vi "PDF_Interface_PDF Protokoll HangUp.vi"(8 "error in (no error)":errorcluster caption="Fehler (Eingang, kein Fehler)", 11 "Save PDF File Path":path) -> (0 "error out":errorcluster caption="Fehler (Ausgang)")   [LabVIEW 2020, in "Hangup Check.lvlib"]
uses:
  Hangup Check.lvlib
  Sprachverwaltung/FGV Aktion Tabelle zerlegen.ctl
  AktionFGV Hangup.ctl
  Seiten/System Einstellungen V2/Aktioen FGV System Konstanten.ctl
  PDF_Interface/PDF Protokoll Standard Kopf Optionen.ctl
  <vilib>/Simplicity AI/SAI_PDF_API/Classes/Context/Controls/SAI_PDF_PDF Details.ctl
  PDF_Interface/PDF Interface Helper/PDFContentType.ctl
  PDF_Interface/PDF Interface Helper/PDFTableContentType.ctl
  PDF_Interface/PDF Interface Helper/PDFResults.ctl
  PDF_Interface/PDF Interface Helper/PDFResultPictures.ctl
  PDF_Interface/PDF Interface Helper/PDFCommentPosition.ctl
  PDF_Interface/PDF Interface Helper/PDFPageBreak.ctl
  PDF_Interface/PDF Interface Helper/PDFTablePictures.ctl
  PDF_Interface/PDF Interface Helper/PDFBemerkung.ctl
  <vilib>/Simplicity AI/SAI_PDF_API/Classes/Context/Controls/SAI_PDF_Text Align.ctl
  <vilib>/Simplicity AI/SAI_PDF_API/Classes/Context/Controls/SAI_PDF_Font.ctl
  <vilib>/Simplicity AI/SAI_PDF_API/Classes/Context/Controls/SAI_PDF_Font Encoding.ctl
  Allgemein/allgemeine Sub-VIs.lvlib
  Seiten/System Einstellungen V2/System Einstellungen V2.lvlib
  Sprachverwaltung/Sprachverwaltung.lvlib
  PDF_Interface/PDF Interface.lvlib
  <vilib>/Simplicity AI/SAI_PDF_API/Classes/Context/Context.lvclass
  PDF_Interface/PDF Interface Helper/PDF Interface Helper.lvlib
  Linearisierung V2/Protokoll/Protokoll.lvlib
panel:
  out "Bestanden":bool caption="Boolesch"
  out "Grenzwert:":string
  out "Nullgas Messwert:":string
  out "Datenerfassungszeit:":string
  out "Nullgas Aufschaltzeit:":string
  out "Analysator:":string
  out "Aufschaltpunkt:":string
  out "Messbereich:":string
  out "Endzeit:":string
  out "Startzeit:":string
  out "Ser.Nr.:":string caption="Serien Nummer:"
  out "Messgerät:":string
  # "Hang - up Check"
  # "ppm"
  # "s"
  # "s"
  # "ppmC3"
  # "ppmC3"
  # "IAG-Industrie Automatisierungsgeschellschaft m.b.H.    l  Industriestraße 2    l    2722Weikersdorf     )+43262221734 7+43262221734655"
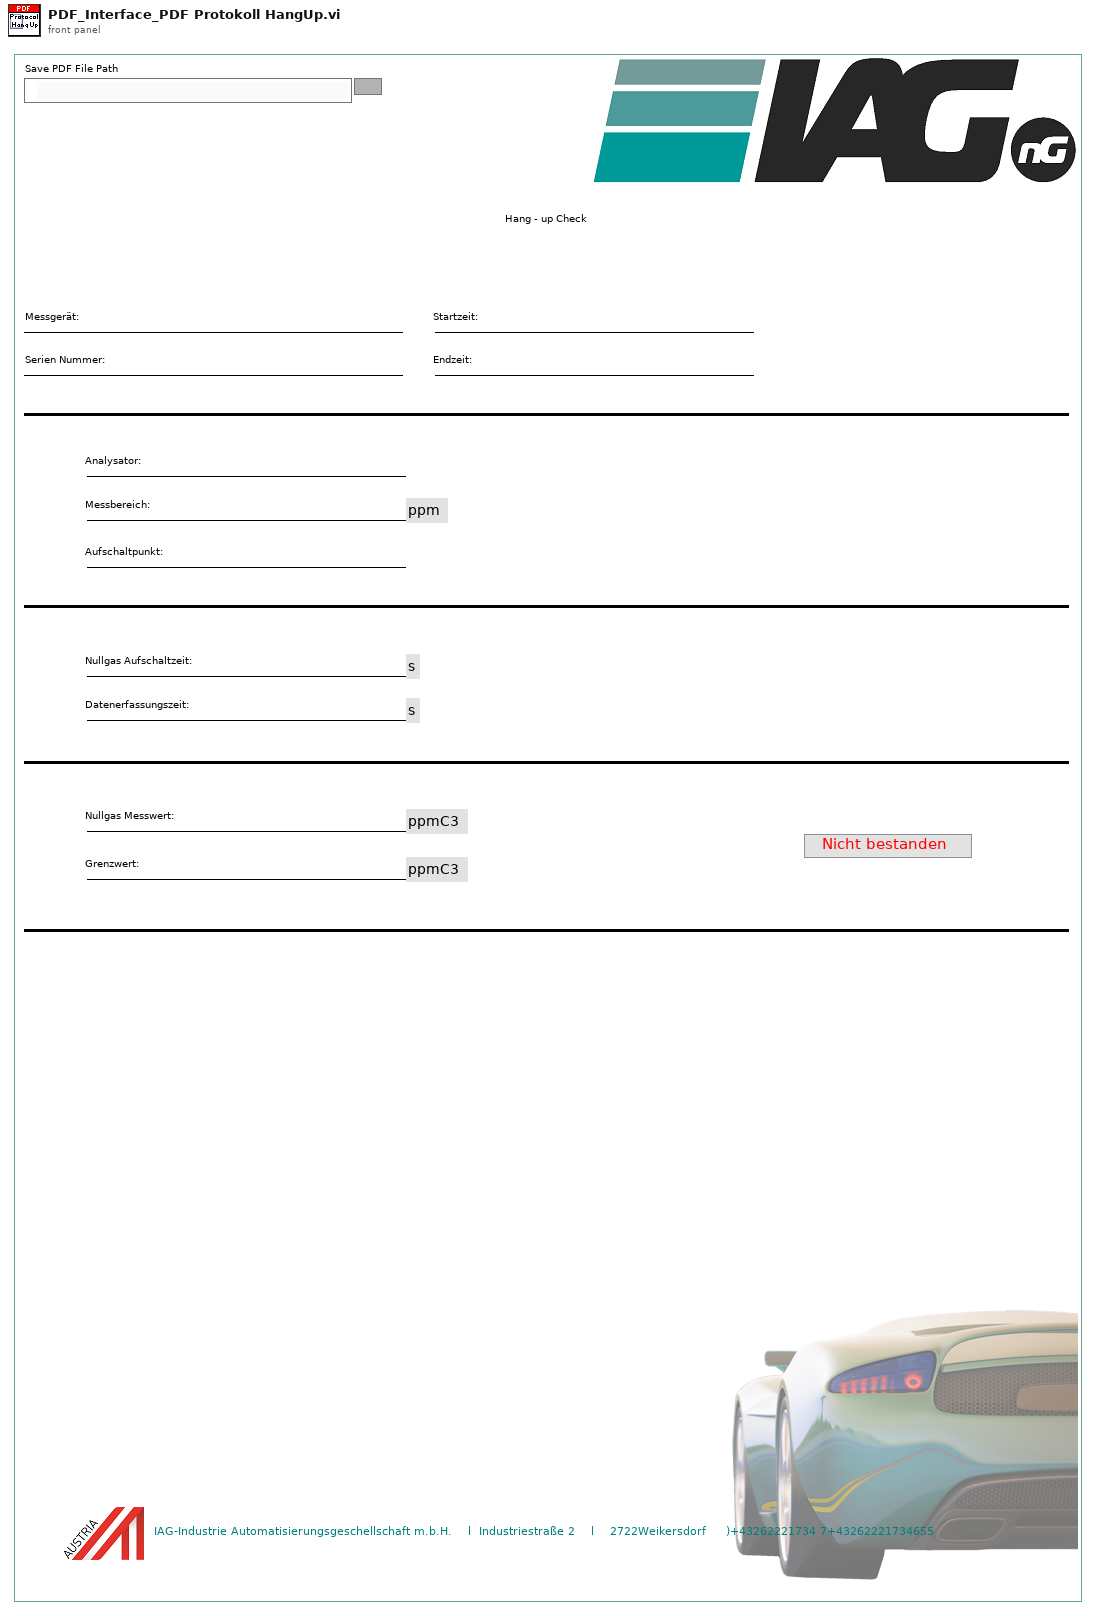
[diagram p1: front panel]
types:
  T1 = typedef "Sprachverwaltung.lvlib/FGV Aktion Tabelle zerlegen.ctl" = enum16{"laden", "vereinzeln", "speichern"}
  T2 = typedef "PDF Interface.lvlib/PDF Protokoll Standard Kopf Optionen.ctl" = cluster{"Analysator":bool, "FT-IR Rezept":bool, "Gasteiler":bool, "Gas Komponente":bool, "Gas Flasche":bool, "LIN Protokoll":bool, "Operator":bool}
  T3 = typedef "System Einstellungen V2.lvlib/Aktioen FGV System Konstanten.ctl" = enum16{"lesen", "laden", "speichern", "Sprache"}
  T4 = typedef "Hangup Check.lvlib/AktionFGV Hangup.ctl" = enum16{"lesen", "Hangup Settings", "Protokoll", "Pfad", "laden", "speichern"}
  T5 = typedef "PDF Interface.lvlib/PDF Interface Helper.lvlib/PDFBemerkung.ctl" = cluster{"Bemerkung Text":string, "Align (Left)":T6, "Add Line Feeds (F:No)":bool, "Font":T7}
  T6 = typedef "SAI_PDF_Toolkit.lvlib/Context.lvclass/SAI_PDF_Text Align.ctl" = i32
  T7 = typedef "SAI_PDF_Toolkit.lvlib/Context.lvclass/SAI_PDF_Font.ctl" = cluster{"Font":string, "Size":i32, "Colour":u32, "Bold":bool, "Italic":bool, "Underline":bool, "Strikethrough":bool, "Font Encoding":T8}
  T8 = typedef "SAI_PDF_Toolkit.lvlib/Context.lvclass/SAI_PDF_Font Encoding.ctl" = enum16{"Cp1252, WinANSI", "IdentityH", "IdentityV", "Cp1250", "Cp1257", "MacRoman"}
  T9 = typedef "PDF Interface.lvlib/PDF Interface Helper.lvlib/PDFResults.ctl" = cluster{"Results":cluster{"Result Text":string, "Result":bool}[], "ResultPictures":T10, "use Pictures":bool, "Image Scale (%)":sgl, "Autoscale? (T)":bool, "Horizontal Align":i32, "Position":i32}
  T10 = typedef "PDF Interface.lvlib/PDF Interface Helper.lvlib/PDFResultPictures.ctl" = cluster{"Yes Ctl Refnum":refnum<vi>, "No Ctl Refnum":refnum<vi>}
  T11 = typedef "PDF Interface.lvlib/PDF Interface Helper.lvlib/PDFTableContentType.ctl" = cluster{"TableHeader":string[], "Table":string[][], "Relative Column Widths (%)":sgl[], "Results":T9, "PositionBemerkung":T12, "PageBreak":T13, "TablePictures":T14, "Horizontal Align":i32}
  T12 = typedef "PDF Interface.lvlib/PDF Interface Helper.lvlib/PDFCommentPosition.ctl" = enum16{"before", "after"}
  T13 = typedef "PDF Interface.lvlib/PDF Interface Helper.lvlib/PDFPageBreak.ctl" = enum16{"none", "before", "after", "after comment"}
  T14 = typedef "PDF Interface.lvlib/PDF Interface Helper.lvlib/PDFTablePictures.ctl" = cluster{"Ctl Refnum In":refnum<vi>[], "RowOrColumn":enum16{"Row", "Column"}, "IndexToInsert":u16, "Image Scale (%)":sgl[], "Autoscale? (T)":bool[], "Horizontal Align":i32}
  T15 = typedef "PDF Interface.lvlib/PDF Interface Helper.lvlib/PDFContentType.ctl" = cluster{"Titel":string, "Header Table":string[][], "Table Array":T11[], "Bemerkungen":T5[]}
  T16 = typedef "SAI_PDF_Toolkit.lvlib/Context.lvclass/SAI_PDF_PDF Details.ctl" = cluster{"Title":string, "Subject":string, "Keywords":string, "Author":string, "Creator":string}
  T17 = cluster{"Header Footer Text Cluster":cluster{"Header Text":string, "Footer Text":string, "Time":string, "Page Number":string}, "PDF Details":T16}
  T18 = typedef "Hangup Check.lvlib/HangupSettings.ctl" = cluster{"Kalibriergas":T19, "Aufschaltpunkt":T19, "Spangas Aufschaltzeit:":sgl, "Nullgas Aufschaltzeit:":sgl, "Datenerfassungszeit:":sgl, "Grenzwert manuell:":sgl, "Grenzwert:":sgl, "Grenze":T19, "Messbereich":T19, "Spankonzentration [ppm]":sgl, "Grenzwert: C1":sgl}
  T19 = typedef "Auswahlfeld.ctl" = u16
  T20 = typedef "Hangup Check.lvlib/Protokoll.ctl" = cluster{"FID Mittelwert 0":sgl, "FID Mittelwert E":sgl, "Messgasdruck Amium":sgl, "Startzeit":timestamp, "Endzeit":timestamp, "Bestanden?":bool}
  T21 = cluster{"Modell":string, "ProjektNummer":string, "Software Version":string, "Seriennummer":string}
  T22 = cluster{"Header Size":i32, "Column Ratio left":sgl[]}
  T23 = typedef "String - Ausgabefeld.ctl" = string
  T24 = cluster{"String - Ausgabefeld":T23, "Bestanden?":bool}
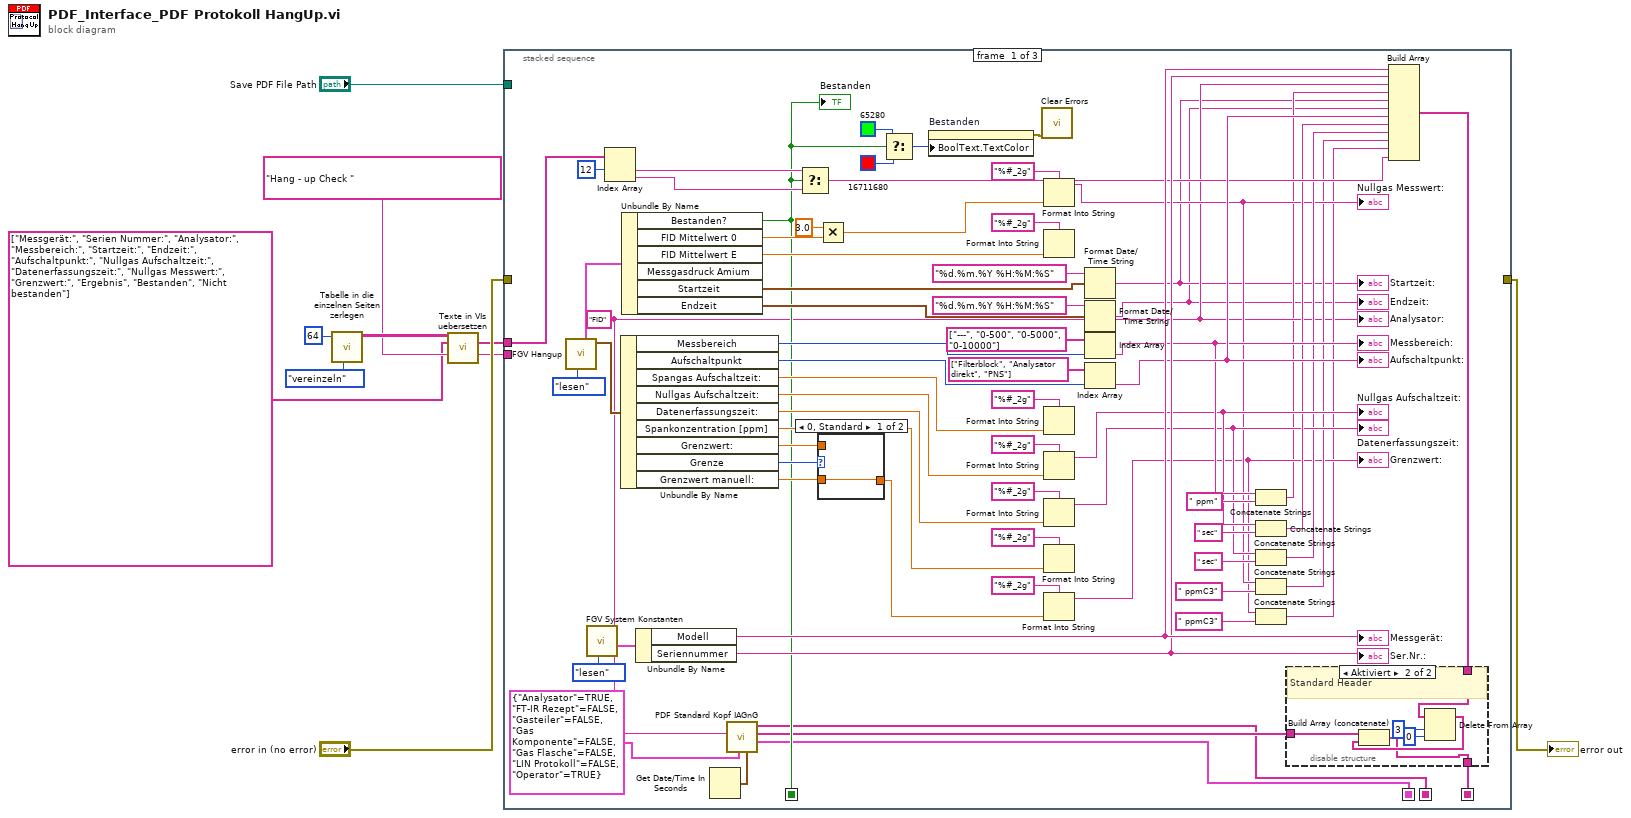
[diagram p0: block diagram]
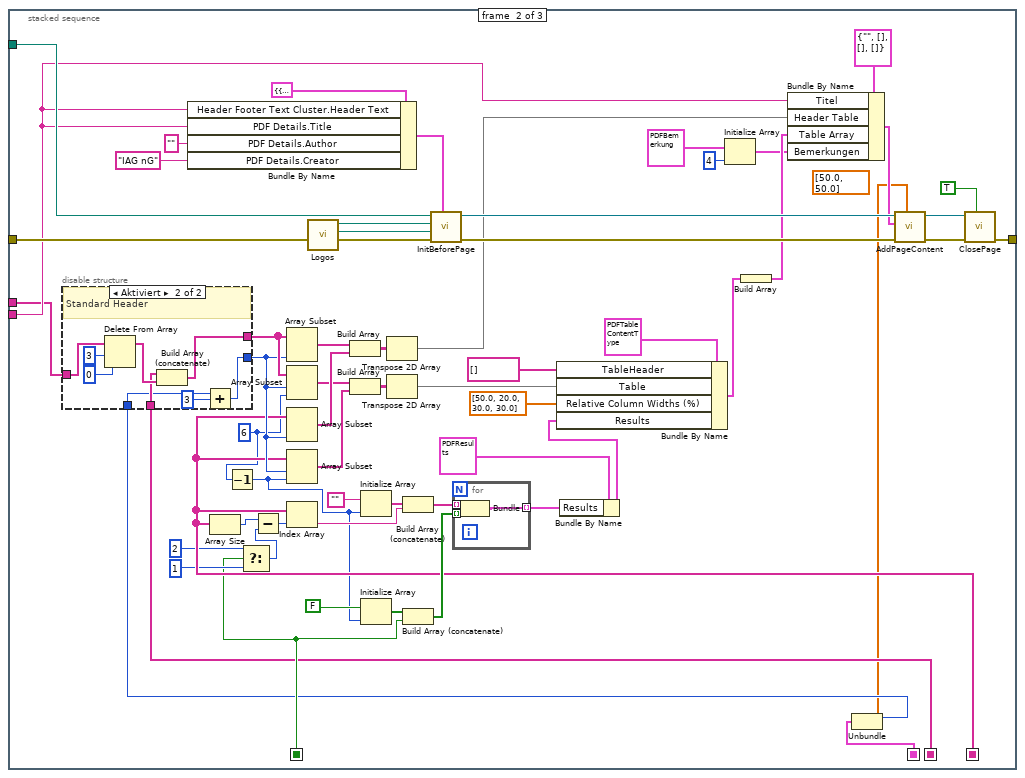
[diagram p4: hidden frame]
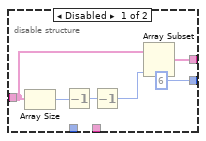
[diagram p5: hidden frame]
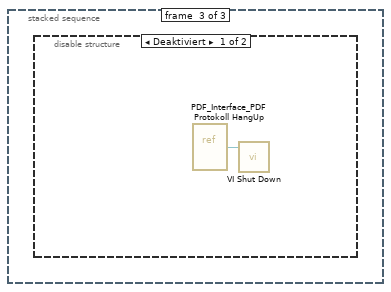
[diagram p6: hidden frame]
diagram:
  n1 = call "Tabelle in die einzelnen Seiten zerlegen.vi"("Aktion"=FGV_Aktion_Tabelle_zerlegen."vereinzeln", "Index (Seite)"=64) -> ("Sprachliste"=w8:string[][])  [unwired: 7 in, 2 out]
  n2 = call "Texte in VIs uebersetzen.vi"("Sprachliste"=w8, "String-Array zum Übersetzen"=string[] ["Messgerät:", "Serien Nummer:", "Analysator:", "Messbereich:", "Startzeit:", "Endzeit:", "Aufschaltpunkt:", "Nullgas Aufschaltzeit:", "Datenerfassungszeit:", "Nullgas Messwert:", "Grenzwert:", "Ergebnis", "Bestanden", "Nicht bestanden"], "String zum Übersetzen"="Hang - up Check ") -> ("String-Array zum Übersetzen"=w2:string[], "String zum Übersetzen"=w1:string)  [unwired: 8 in, 3 out]
  n3 = stacked-sequence {
    seq-local: [w36 _ _] -> [_ w97 _]
    seq-local: [w20 _ _] -> [_ w100 _]
    seq-local: [w16 _ _] -> [_ w92 _]
    seq-local: [w17 _ _] -> [_ w94 _]
    tunnel: "Save PDF File Path" -> [_ w105 _]
    tunnel: "error in (no error)" -> [_ w104 _]
    tunnel: [_ w103 _] -> w3
    tunnel: w2 -> [w40 w101 _]
    tunnel: w1 -> [_ w102 _]
    frame #0 {
      w15 = "FID" ("Analysator:")
      n4 = call "FGV Hangup.vi"("Aktion"=AktionFGV_Hangup."lesen") -> ("Hangup Settings"=w78:T18, "Protokoll"=w79:T20)  [unwired: 6 in, 3 out]
      n5 = call "FGV System Konstanten.vi"("Aktionen"=Aktioen_FGV_System_Konstanten."lesen") -> ("Cluster out"=w76:T21)  [unwired: 6 in, 4 out]
      n6 = Index Array(array=w40, index #1=12 ("Index")) -> (element #1=w39:string, element #2=w38:string)  [unwired: 1 in]
      n7 = Unbundle By Name(w78) -> ("Messbereich"=w69:T19, "Aufschaltpunkt"=w68:T19, "Spangas Aufschaltzeit:"=w66:sgl, "Nullgas Aufschaltzeit:"=w64:sgl, "Datenerfassungszeit:"=w62:sgl, "Spankonzentration [ppm]"=w60:sgl, "Grenzwert:"=w57:sgl, "Grenze"=w59:T19, "Grenzwert manuell:"=w58:sgl)
      n8 = Unbundle By Name(w79) -> ("Bestanden?"=w36:bool, "FID Mittelwert 0"=w51:sgl, "FID Mittelwert E"=w53:sgl, "Startzeit"=w73:timestamp, "Endzeit"=w72:timestamp)  [unwired: 1 out]
      "Bestanden" <- w36
      n9 = Unbundle By Name(w76) -> ("Modell"=w44:string, "Seriennummer"=w43:string)
      "Messgerät:" <- w44
      "Ser.Nr.:" <- w43
      n10 = Get Date/Time In Seconds() -> (seconds since 1Jan1904=w11:timestamp)
      n11 = call "PDF Standard Kopf IAGnG.vi"("Zeitstempel"=w11, "Oprtionen Cluster"=T2 {"Analysator"=TRUE, "FT-IR Rezept"=FALSE, "Gasteiler"=FALSE, "Gas Komponente"=FALSE, "Gas Flasche"=FALSE, "LIN Protokoll"=FALSE, "Operator"=TRUE}, "Analysator"=w15) -> ("Size Cluster"=w16:T22, "Header Values"=w18:T23[], "Header Labels"=w17:string[])  [unwired: 5 in, 1 out]
      n12 = Select(t=w39, s=w36, f=w38) -> (s? t:f=w37:string)
      n13 = Multiply(x=sgl 3.0 ("y"), y=w51) -> (x*y=w46:sgl)
      n14 = case shown="0, Standard" w59 {
        tunnel: w58 -> [w88 _]
        tunnel: [w88 w89] -> w56
        tunnel: w57 -> [_ w89]
        frame 0, Default {
        }
        frame 1 {
        }
      }
      n15 = Select(t=u32 65280, s=w36, f=u32 16711680) -> (s? t:f=w48:u32)
      n16 = property on="Bestanden" class="Bool. (strikt)"("BoolText.TextColor"=w48) -> (error out=w47:errorcluster)  [unwired: 2 in, 1 out]
      n17 = call <vilib>:"Clear Errors.vi"("error in (no error)"=w47) -> ()  [unwired: 5 in, 2 out]
      n18 = Format Into String(format string="%#_2g" ("Format-String"), w46) -> (resulting string=w25:string)  [unwired: 2 in, 1 out]
      "Nullgas Messwert:" <- w25
      n19 = Format Into String(format string="%#_2g" ("Format-String"), w53) -> ()  [unwired: 2 in, 2 out]
      n20 = Format Into String(format string="%#_2g" ("Format-String"), w66) -> ()  [unwired: 2 in, 2 out]
      n21 = Format Into String(format string="%#_2g" ("Format-String"), w64) -> (resulting string=w29:string)  [unwired: 2 in, 1 out]
      "Nullgas Aufschaltzeit:" <- w29
      n22 = Format Into String(format string="%#_2g" ("Format-String"), w62) -> (resulting string=w27:string)  [unwired: 2 in, 1 out]
      "Datenerfassungszeit:" <- w27
      n23 = Format Into String(format string="%#_2g" ("Format-String"), w60) -> ()  [unwired: 2 in, 2 out]
      n24 = Format Into String(format string="%#_2g" ("Format-String"), w56) -> (resulting string=w23:string)  [unwired: 2 in, 1 out]
      "Grenzwert:" <- w23
      n25 = Format Date/Time String(time format string (%c)="%d.%m.%Y %H:%M:%S" ("Zeitformatierungs-String (%c)"), seconds (now)=w73) -> (date/time string=w13:string)  [unwired: 1 in]
      "Startzeit:" <- w13
      n26 = Format Date/Time String(time format string (%c)="%d.%m.%Y %H:%M:%S" ("Zeitformatierungs-String (%c)"), seconds (now)=w72) -> (date/time string=w12:string)  [unwired: 1 in]
      "Endzeit:" <- w12
      n27 = Index Array(array=string[] ["---", "0-500", "0-5000", "0-10000"], index=w69) -> (element=w30:string)
      "Messbereich:" <- w30
      n28 = Index Array(array=string[] ["Filterblock", "Analysator direkt", "PNS"], index=w68) -> (element=w42:string)
      "Aufschaltpunkt:" <- w42
      n29 = Concatenate Strings(w30, " ppm" ("String")) -> (w14:string)
      n30 = Concatenate Strings(w29, " sec" ("String")) -> (w28:string)
      n31 = Concatenate Strings(w27, " sec" ("String")) -> (w26:string)
      n32 = Concatenate Strings(w25, " ppmC3" ("String")) -> (w24:string)
      n33 = Concatenate Strings(w23, " ppmC3" ("String")) -> (w22:string)
      n34 = Build Array(w44, w43, w15, w14, w13, w12, w42, w28, w26, w24, w22, w37) -> (w19:string[])
      n35 = disable-structure shown="Aktiviert" {
        disable-tunnel: [w81 w84] -> w20
        disable-tunnel: w19 -> [w81 w87]
        disable-tunnel: w18 -> [_ w86]
        frame Disabled {
        }
        frame Enabled {
          # "Standard Header"
          n36 = Delete From Array(array=w87, length=3 ("Länge"), index=0 ("Index")) -> (array with subset deleted=w85:string[])  [unwired: 1 out]
          n37 = Build Array (concatenate)(w86, w85) -> (w84:T23[])
        }
      }
      "Analysator:" <- w15
    }
    frame #1 {
      w93 = 6 ("Länge")
      (unwired) sgl[] [50.0, 50.0] ("Column Ratio left")
      n38 = Bundle By Name(cluster=T17 {"Header Footer Text Cluster"={"Header Text"="Protokoll XYZ", "Footer Text"="IAG nG", "Time"="<TIMESTAMP yyyy-MM-dd>", "Page Number"="Page <P> of <PT>"}, "PDF Details"={"Title"="Test PDF", "Subject"="Versa Tabasco", "Keywords"="", "Author"="RIW", "Creator"="IAG"}} ("Info"), "Header Footer Text Cluster.Header Text"=w102, "PDF Details.Title"=w102, "PDF Details.Author"="", "PDF Details.Creator"="IAG nG") -> (w138:T17)
      n39 = Array Size(array=w100) -> (size(s)=w131:i32)
      n40 = Decrement(x=w93) -> (x-1=w95:i32)
      n41 = Select(t=2 ("Länge"), s=w97, f=1 ("Länge")) -> (s? t:f=w96:i32)
      n42 = Subtract(x=w131, y=w96) -> (x-y=w123:i32)
      n43 = Index Array(array=w100, index=w123) -> (element=w128:T23)
      n44 = call "Logos.vi"() -> ("Footer Image File Path"=w147:path, "Header Image File Path"=w148:path)  [unwired: 8 in, 2 out]
      n45 = Initialize Array("", w95) -> (w129:string[])
      n46 = Initialize Array(FALSE, w95) -> (w121:bool[])
      n47 = Build Array (concatenate)(w129, w128) -> (w120:T23[])
      n48 = Build Array (concatenate)(w121, w97) -> (w119:bool[])
      n49 = call "InitBeforePage.vi"("Info"=w138, "Fehler (Eingang, kein Fehler)"=w104, "Footer Image File Path"=w147, "Header Image File Path"=w148, "Path (Dialog if Empty)"=w105) -> ("Fehler (Ausgang)"=w146:errorcluster, "Context (Ausgang)"=w145:refnum<class "Context.lvclass">)  [unwired: 5 in]
      n50 = for {
        tunnel: w120 -> [w166] mode=indexing
        tunnel: w119 -> [w165] mode=indexing
        tunnel: [w164] -> w107 mode=indexing
        n51 = Bundle("String - Ausgabefeld"=w166, "Bestanden?"=w165) -> (w164:T24)  [unwired: 1 in]
      }
      n52 = Bundle By Name(cluster=T9 {"Results"=[], "ResultPictures"={"Yes Ctl Refnum"=refnum, "No Ctl Refnum"=refnum}, "use Pictures"=FALSE, "Image Scale (%)"=100.0, "Autoscale? (T)"=TRUE, "Horizontal Align"=3, "Position"=0} ("Results"), "Results"=w107) -> (w108:T9)
      n53 = Initialize Array(T5 {"Bemerkung Text"="", "Align (Left)"=0, "Add Line Feeds (F:No)"=FALSE, "Font"={"Font"="Arial", "Size"=10, "Colour"=0, "Bold"=FALSE, "Italic"=FALSE, "Underline"=FALSE, "Strikethrough"=FALSE, "Font Encoding"=enum."Cp1252, WinANSI"}} ("Bemerkung"), 4 ("Dimensionsgröße")) -> (w111:T5[])
      n54 = Unbundle(w92) -> ("Header Size"=w91:i32, "Column Ratio left"=w90:sgl[])
      n55 = disable-structure shown="Aktiviert" {
        disable-tunnel: [w151 w158] -> w133
        disable-tunnel: [6 ("Länge") w155] -> w132
        disable-tunnel: w101 -> [w149 w163]
        disable-tunnel: w94 -> [_ w159]
        disable-tunnel: w91 -> [_ w157]
        frame Disabled {
          n56 = Array Size(array=w149) -> (size(s)=w154:i32)
          n57 = Decrement(x=w154) -> (x-1=w153:i32)
          n58 = Decrement(x=w153) -> (x-1=w152:i32)
          n59 = Array Subset(array=w149, length=w152) -> (w151:string[])  [unwired: 1 in]
        }
        frame Enabled {
          # "Standard Header"
          n60 = Delete From Array(array=w163, length=3 ("Länge"), index=0 ("Index")) -> (array with subset deleted=w160:string[])  [unwired: 1 out]
          n61 = Build Array (concatenate)(w159, w160) -> (w158:string[])
          n62 = Add(x=w157, y=3) -> (x+y=w155:i32)
        }
      }
      n63 = Array Subset(array=w133, length=w132) -> (w136:string[])  [unwired: 1 in]
      n64 = Array Subset(array=w133, index=w132, length=w93) -> (w126:string[])
      n65 = Array Subset(array=w100, length=w132) -> (w135:T23[])  [unwired: 1 in]
      n66 = Array Subset(array=w100, index=w132, length=w95) -> (w125:T23[])
      n67 = Build Array(w136, w135) -> (w134:T23[][])
      n68 = Build Array(w126, w125) -> (w124:T23[][])
      n69 = Transpose 2D Array(2D array=w134) -> (transposed array=w114:T23[][])
      n70 = Transpose 2D Array(2D array=w124) -> (transposed array=w113:T23[][])
      n71 = Bundle By Name(cluster=T11 {"TableHeader"=[], "Table"=[], "Relative Column Widths (%)"=[], "Results"={"Results"=[], "ResultPictures"={"Yes Ctl Refnum"=refnum, "No Ctl Refnum"=refnum}, "use Pictures"=FALSE, "Image Scale (%)"=0.0, "Autoscale? (T)"=FALSE, "Horizontal Align"=0, "Position"=0}, "PositionBemerkung"=enum."before", "PageBreak"=enum."none", "TablePictures"={"Ctl Refnum In"=[], "RowOrColumn"=enum."Row", "IndexToInsert"=0, "Image Scale (%)"=[], "Autoscale? (T)"=[], "Horizontal Align"=0}, "Horizontal Align"=0} ("Table Array"), "TableHeader"=string[] [], "Table"=w113, "Relative Column Widths (%)"=sgl[] [50.0, 20.0, 30.0, 30.0], "Results"=w108) -> (w117:T11)
      n72 = Build Array(w117) -> (w116:T11[])
      n73 = Bundle By Name(cluster=T15 {"Titel"="", "Header Table"=[], "Table Array"=[], "Bemerkungen"=[]} ("Content"), "Titel"=w102, "Header Table"=w114, "Table Array"=w116, "Bemerkungen"=w111) -> (w115:T15)
      n74 = call "AddPageContent.vi"("Column Ratio left"=w90, "error in"=w146, "Content"=w115, "Context (Eingang)"=w145) -> ("error out"=w144:errorcluster, "Context (Ausgang)"=w143:refnum<class "Context.lvclass">)  [unwired: 6 in]
      n75 = call "ClosePage.vi"("popup viewer"=TRUE, "Fehler (Eingang, kein Fehler)"=w144, "Context (Eingang)"=w143) -> ("Fehler (Ausgang)"=w103:errorcluster)  [unwired: 8 in]
    }
    frame #2 {
      n76 = disable-structure shown="Deaktiviert" {
        frame Disabled {
          n77 = vi-ref "PDF_Interface_PDF Protokoll HangUp.vi"() -> (w167:refnum<vi>)
          n78 = call "VI Shut Down.vi"("VI Referenz"=w167) -> ()  [unwired: 11 in]
        }
        frame Enabled {
        }
      }
    }
  }
  "error out" <- w3
